vi "CONEX-LDS Set Low Power Threshold v2.vi"(9 "Negative limit (left)":dbl, 11 "Connection Cluster in":T1) -> (3 "Connection Cluster out":T1)   [LabVIEW 2010]
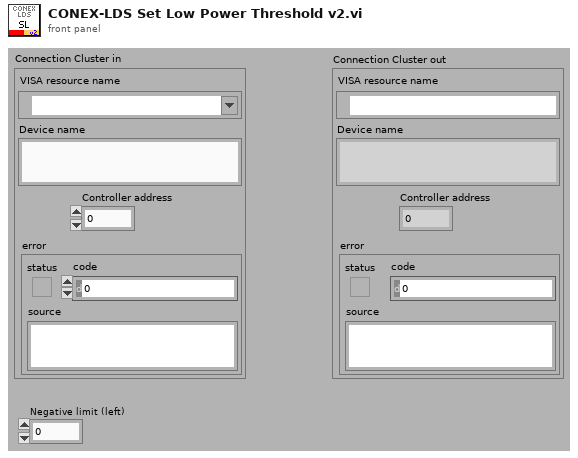
[diagram p1: front panel]
types:
  T1 = cluster{"VISA resource name":refnum<visa-resource-name>, "Device name":string, "Controller address":i32, "error":errorcluster}
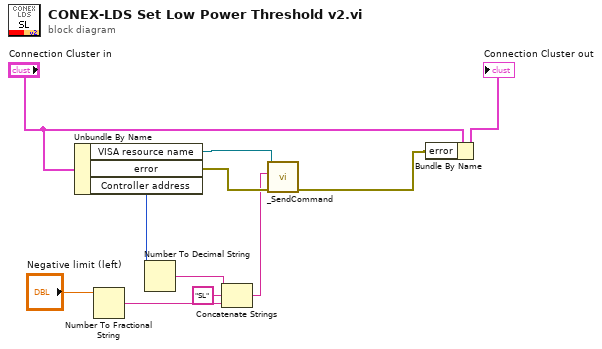
[diagram p0: block diagram]
diagram:
  n1 = Unbundle By Name("Connection Cluster in") -> ("VISA resource name"=w7:refnum<visa-resource-name>, "error"=w5:errorcluster, "Controller address"=w1:i32)
  n2 = Number To Fractional String(number="Negative limit (left)") -> (F-format string=w8:string)  [unwired: 3 out]
  n3 = Number To Decimal String(number=w1) -> (decimal integer string=w11:string)  [unwired: 1 out]
  n4 = Concatenate Strings(w11, "SL" ("strCommand"), w8) -> (w2:string)
  n5 = call <userlib>:"_SendCommand.vi"("error in"=w5, "Command"=w2, "Instrument Channel"=w7) -> ("error out"=w6:errorcluster)  [unwired: 7 in, 1 out]
  n6 = Bundle By Name(cluster="Connection Cluster in", "error"=w6) -> (→"Connection Cluster out":T1)
